vi "Resize Message String & Dialog Window.vi"(6 "Max Number of Lines":i32, 8 "Error In":errorcluster, 9 "Message":string, 10 "Controls & Indicators":T1, 11 "VI Refnum":refnum<vi>) -> (0 "Error Out":errorcluster, 3 "VI Refnum out":refnum<vi>)   [LabVIEW 2019]
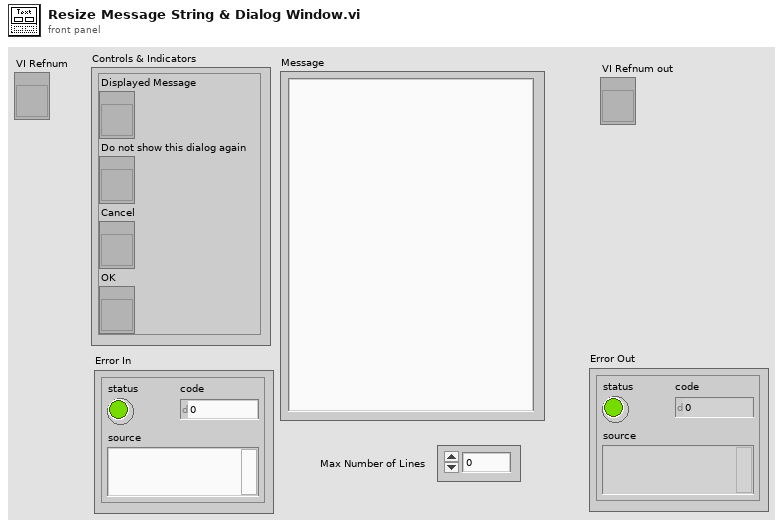
[diagram p1: front panel]
types:
  T1 = cluster{"Displayed Message":refnum<vi>, "Do not show this dialog again":refnum<vi>, "Cancel":refnum<vi>, "OK":refnum<vi>}
  T2 = typedef "LVRectTypeDef.ctl" = cluster{"Left":i16, "Top":i16, "Right":i16, "Bottom":i16}
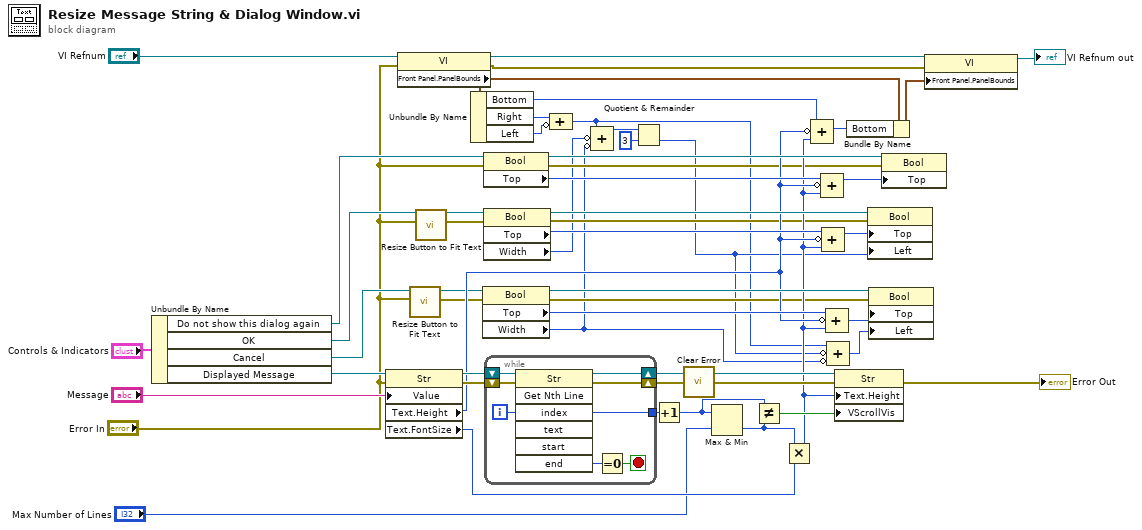
[diagram p0: block diagram]
diagram:
  n1 = Unbundle By Name("Controls & Indicators") -> ("Do not show this dialog again"=w32:refnum<vi>, "OK"=w4:refnum<vi>, "Cancel"=w28:refnum<vi>, "Displayed Message"=w39:refnum<vi>)
  n2 = property class="Str"(reference=w39, error in="Error In", "Value"="Message") -> (reference out=w53:refnum<vi>, error out=w52:errorcluster, "Text.Height"=w22:u32, "Text.FontSize"=w49:u32)
  n3 = property class="VI"(reference="VI Refnum", error in="Error In") -> (reference out=w35:refnum<vi>, error out=w34:errorcluster, "Front Panel.PanelBounds"=w37:T2)
  n4 = call "Resize Button to Fit Text.vi"("error in (no error)"="Error In", "Boolean in"=w28) -> ("error out"=w5:errorcluster, "Boolean out"=w6:refnum<vi>)  [unwired: 8 in]
  n5 = call "Resize Button to Fit Text.vi"("error in (no error)"="Error In", "Boolean in"=w4) -> ("error out"=w1:errorcluster, "Boolean out"=w3:refnum<vi>)  [unwired: 8 in]
  n6 = Unbundle By Name(w37) -> ("Bottom"=w38:i16, "Right"=w10:i16, "Left"=w9:i16)
  n7 = property class="Bool"(reference=w6, error in=w5) -> (reference out=w26:refnum<vi>, error out=w16:errorcluster, "Top"=w23:i32, "Width"=w12:u32)
  n8 = property class="Bool"(reference=w32, error in="Error In") -> (reference out=w30:refnum<vi>, error out=w18:errorcluster, "Top"=w31:i32)
  n9 = property class="Bool"(reference=w3, error in=w1) -> (reference out=w27:refnum<vi>, error out=w17:errorcluster, "Top"=w25:i32, "Width"=w15:u32)
  n10 = while {
    shift-right: [w59] -> w47
    shift-left: w52 -> [w60]
    shift-right: [w58] -> w48
    shift-left: w53 -> [w61]
    tunnel: [w56] -> w50
    i -> [w56]
    stop <- w55 stop-if-true
    n11 = invoke class="Str" method="Get Nth Line"(reference=w61, error in=w60, "index"=w56) -> (reference out=w58:refnum<vi>, error out=w59:errorcluster, "end"=w57:u32)  [unwired: 4 in, 4 out]
    n12 = Equal To 0?(x=w57) -> (x = 0?=w55:bool)
  }
  n13 = Compound Arithmetic op=ADD(w10, invert w9) -> (w8:i16)
  n14 = Compound Arithmetic op=ADD(w8, invert w15, invert w12) -> (w14:u32)
  n15 = Quotient & Remainder(x=w14, y=u32 3) -> (floor(x/y)=w11:u32)  [unwired: 1 out]
  n16 = Increment(x=w50) -> (x+1=w43:i32)
  n17 = call "Clear Error.vi"("Error In"=w47) -> ("no Error Out"=w45:errorcluster)  [unwired: 8 in]
  n18 = Max & Min(x=w43, y="Max Number of Lines") -> (min(x,y)=w44:i32)  [unwired: 1 out]
  n19 = Not Equal?(x=w43, y=w44) -> (x != y?=w42:bool)
  n20 = Multiply(x=w44, y=w49) -> (x*y=w21:u32)
  n21 = Compound Arithmetic op=ADD(w38, invert w22, w21) -> (w36:u32)
  n22 = Compound Arithmetic op=ADD(w31, invert w22, w21) -> (w29:u32)
  n23 = Compound Arithmetic op=ADD(w25, invert w22, w21) -> (w24:u32)
  n24 = Compound Arithmetic op=ADD(w23, invert w22, w21) -> (w20:u32)
  n25 = Compound Arithmetic op=ADD(w8, invert w11, invert w12) -> (w7:u32)
  n26 = property class="Str"(reference=w48, error in=w45, "Text.Height"=w21, "VScrollVis"=w42) -> (error out=→"Error Out":errorcluster)  [unwired: 1 out]
  n27 = Bundle By Name(cluster=w37, "Bottom"=w36) -> (w33:T2)
  n28 = property class="Bool"(reference=w27, error in=w17, "Top"=w24, "Left"=w11) -> ()  [unwired: 2 out]
  n29 = property class="Bool"(reference=w26, error in=w16, "Top"=w20, "Left"=w7) -> ()  [unwired: 2 out]
  n30 = property class="Bool"(reference=w30, error in=w18, "Top"=w29) -> ()  [unwired: 2 out]
  n31 = property class="VI"(reference=w35, error in=w34, "Front Panel.PanelBounds"=w33) -> (reference out=→"VI Refnum out":refnum<vi>)  [unwired: 1 out]
